vi "Read Attributes.vi"(11 "Return Device DER_Info Msg":refnum<class "Return Device DER_Info Msg.lvclass">) -> (2 "Payload":cluster{"DER_Info":T1})   [LabVIEW 2016, in "Return Device DER_Info Msg.lvclass"]
uses:
  Return Device DER_Info Msg.lvclass
  <vilib>/ORNL/CSEISMIC DDS/CSEISMIC DDS Base/Data Types/DER_Info.ctl
  <vilib>/ORNL/CSEISMIC DDS/CSEISMIC DDS Base/Data Types/Controls/DeviceID.ctl
  Return Device DER_Info Msg.lvclass/Return Device DER_Info Msg.ctl
  <vilib>/ORNL/CSEISMIC DDS/CSEISMIC DDS Base/CSEISMIC DDS.lvclass
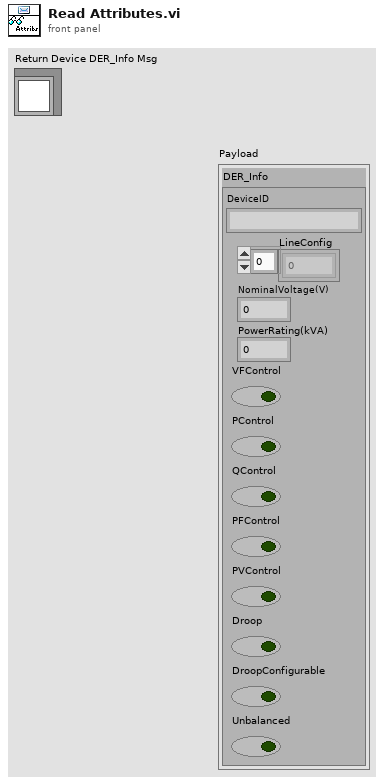
[diagram p1: front panel]
types:
  T1 = typedef "CSEISMIC DDS.lvlib/CSEISMIC DDS.lvclass/DER_Info.ctl" = cluster{"DeviceID":T2, "LineConfig":u8[], "NominalVoltage(V)":dbl, "PowerRating(kVA)":dbl, "VFControl":bool, "PControl":bool, "QControl":bool, "PFControl":bool, "PVControl":bool, "Droop":bool, "DroopConfigurable":bool, "Unbalanced":bool}
  T2 = typedef "CSEISMIC DDS.lvlib/CSEISMIC DDS.lvclass/DeviceID.ctl" = string
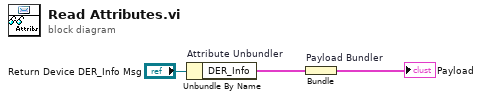
[diagram p0: block diagram]
diagram:
  n1 = Unbundle By Name "Attribute Unbundler"("Return Device DER_Info Msg") -> ("DER_Info"=w1:T1)
  n2 = Bundle "Payload Bundler"("DER_Info"=w1) -> (→"Payload":cluster{"DER_Info":T1})  [unwired: 1 in]
